vi "close methods.vi"(8 "error in (no error)":errorcluster, 11 "Variant":variant) -> (0 "error out":errorcluster)   [LabVIEW 2017]
uses:
  <vilib>/NI/JSON Support for LabVIEW/JSON Value/JSON Value.lvclass
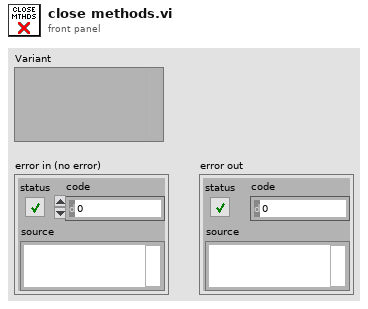
[diagram p1: front panel]
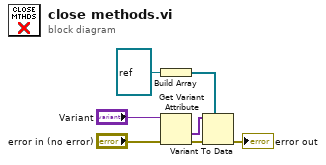
[diagram p0: block diagram]
diagram:
  n1 = Build Array(refnum<vi> refnum ("type specifier VI Refnum (for type only)")) -> (w4:refnum<vi>[])
  n2 = Get Variant Attribute(Variant="Variant", error in="error in (no error)") -> (values=w2:variant[], error out=w5:errorcluster)  [unwired: 2 in, 2 out]
  n3 = Variant To Data(error in=w5, type=w4, Variant=w2) -> (error out=→"error out":errorcluster)  [unwired: 1 out]
